vi "Delete Section.vi"(4 "Return deleted section names? [F]":bool, 7 "Section name":string, 8 "error in (no error)":errorcluster, 10 "Use Regex? [F]":bool, 11 "Carya Config in":refnum<class "Carya Config.lvclass">) -> (0 "error out":errorcluster, 2 "Section names":string[](array[string]), 3 "Carya Config out":refnum<class "Carya Config.lvclass">)   [LabVIEW 2013, in "Carya Config.lvclass"]
doc: "Copyright 2018, Carya Automatisering, Wiebe Walstra."
uses:
  Carya Config.lvclass
  CConfig Object/Delete Query/Delete Query.lvclass
  CConfig Object/Data.ctl
  CConfig Object/Add Results Query/Add Results Query.lvclass
  CConfig Object/CConfig Object.lvclass
  CConfig Object/Composite Query/Composite Query.lvclass
  CConfig Object/Loop Query/Match Query/Match Query.lvclass
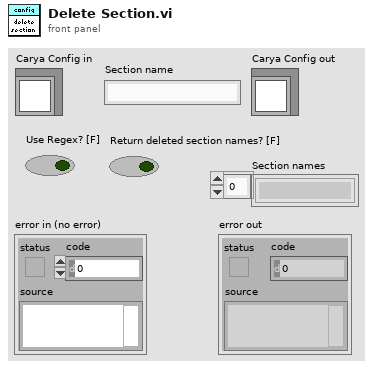
[diagram p1: front panel]
types:
  T1 = typedef "CConfig Object.lvclass/Data.ctl" = enum16{"pre", "name", "middle", "value", "post", "newline", "persistant", "tagged", "type"}
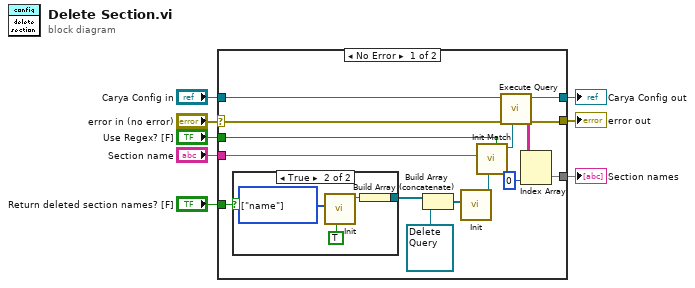
[diagram p0: block diagram]
diagram:
  n1 = case shown="No Error" "error in (no error)" {
    selector: "error in (no error)" -> [w18 w29]
    tunnel: [w19 w29] -> w7
    tunnel: [w20 w28] -> w5
    tunnel: "Carya Config in" -> [w23 w28]
    tunnel: "Section name" -> [w22 _]
    tunnel: "Use Regex? [F]" -> [w11 _]
    tunnel: [w21 _] -> w2
    tunnel: "Return deleted section names? [F]" -> [w9 _]
    frame No Error {
      n2 = case shown="True" w9 {
        tunnel: [_ w24] -> w15
        frame False {
        }
        frame True {
          w25 = T1[] [enum."name"] items=["pre", "name", "middle", "value", "post", "newline", "persistant", "tagged", "type"] ("Data")
          n3 = call "Init.vi"("Concatenate\\Build [T, Concatenate]"=TRUE ("Concatenate\\Build [T, Concatenate]"), "Data [name]"=w25) -> ("Find First Query out"=w26:refnum<class "Add Results Query.lvclass">)  [unwired: 8 in, 1 out]
          n4 = Build Array(w26) -> (w24:refnum<class "Add Results Query.lvclass">[])
        }
      }
      n5 = Build Array (concatenate)(w15, refnum<class "Delete Query.lvclass"> refnum ("Delete Query.lvclass")) -> (w12:refnum<class "CConfig Query.lvclass">[])
      n6 = call "Init.vi"("Queries"=w12) -> ("Step In Query out"=w13:refnum<class "CConfig Query.lvclass">)  [unwired: 9 in, 1 out]
      n7 = call "Init Match.vi"("Regex [F]"=w11, "Found"=w13, "Data"=w22) -> ("Find First Query out"=w10:refnum<class "Loop Query.lvclass">)  [unwired: 7 in, 1 out]
      n8 = call-dynamic "Execute Query.vi"("Config Query in"=w10, "error in (no error)"=w18, "Carya Config in"=w23) -> ("error out"=w19:errorcluster, "Results"=w16:string[][], "Carya Config out"=w20:refnum<class "Carya Config.lvclass">)  [unwired: 4 in, 2 out]
      n9 = Index Array(array=w16, index (col)=0 ("disabled index (col)")) -> (element=w21:string[])  [unwired: 1 in]
    }
    frame Error {
    }
  }
  "error out" <- w7
  "Carya Config out" <- w5
  "Section names" <- w2
